vi "CliSetConnectionParams.vi"(0 "ref in":u64, 5 "Address":string, 7 "LocalTSAP":u16, 9 "RemoteTSAP":u16, 11 "error in (no error)":errorcluster) -> (4 "ref out":u64, 6 "Result":i32, 15 "error out":errorcluster)   [LabVIEW 2020, in "Snap7.lvlib"]
uses:
  Snap7.lvlib
  windows/lv_snap7.dll
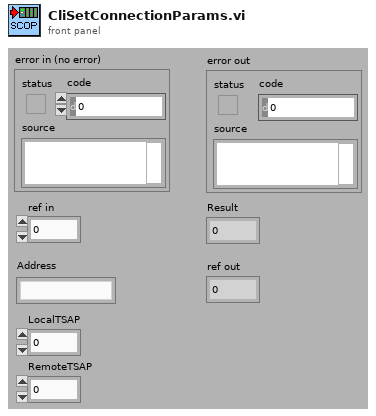
[diagram p1: front panel]
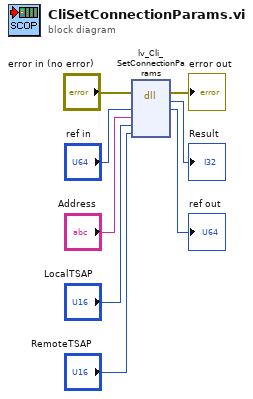
[diagram p0: block diagram]
diagram:
  n1 = dll-call lib="PTH2fabs CUsersFeng项目HLCEPS300-2性能试验台SourcesSnap7libwindowslv_snap7.dll" fn="lv_Cli_SetConnectionParams"(error in="error in (no error)", "Client"="ref in", "Address"="Address", "LocalTSAP"="LocalTSAP", "RemoteTSAP"="RemoteTSAP") -> (error out=→"error out":errorcluster, "return type"=→"Result":i32, "Client"=→"ref out":u64)  [unwired: 5 in, 1 out]
